vi "Relay_On_While_Running.vi"() -> ()   [LabVIEW 2022 SP3]
uses:
  <vilib>/Instr/_visa.llb/VISA Configure Serial Port (Instr).vi
panel:
  out "Controller Feedback":string
  out "Command Sent":string
  in  "VISA resource name":refnum<visa-resource-name>
  in  "Left":bool
  in  "Down":bool
  in  "Up":bool
  in  "Right":bool
  in  "Adjustor Number":dbl format="%0#3_4p"
  in  "Emergency Stop":bool
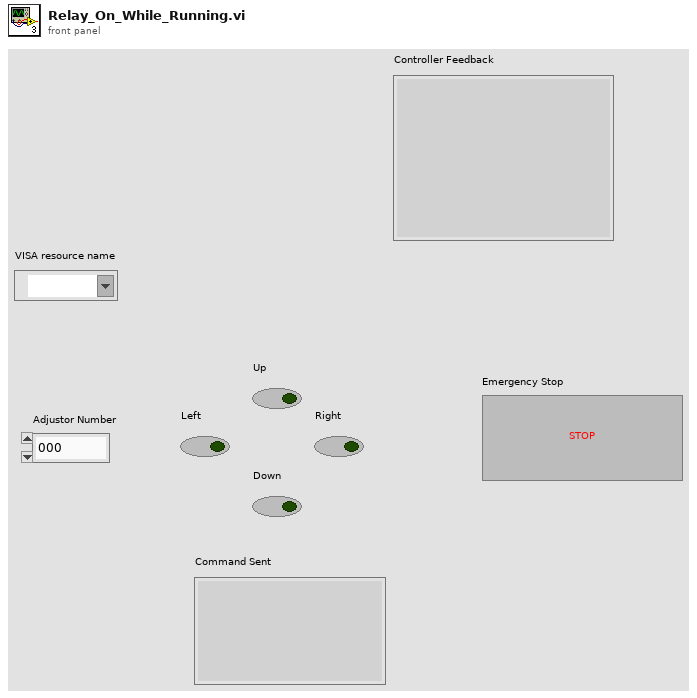
[diagram p1: front panel]
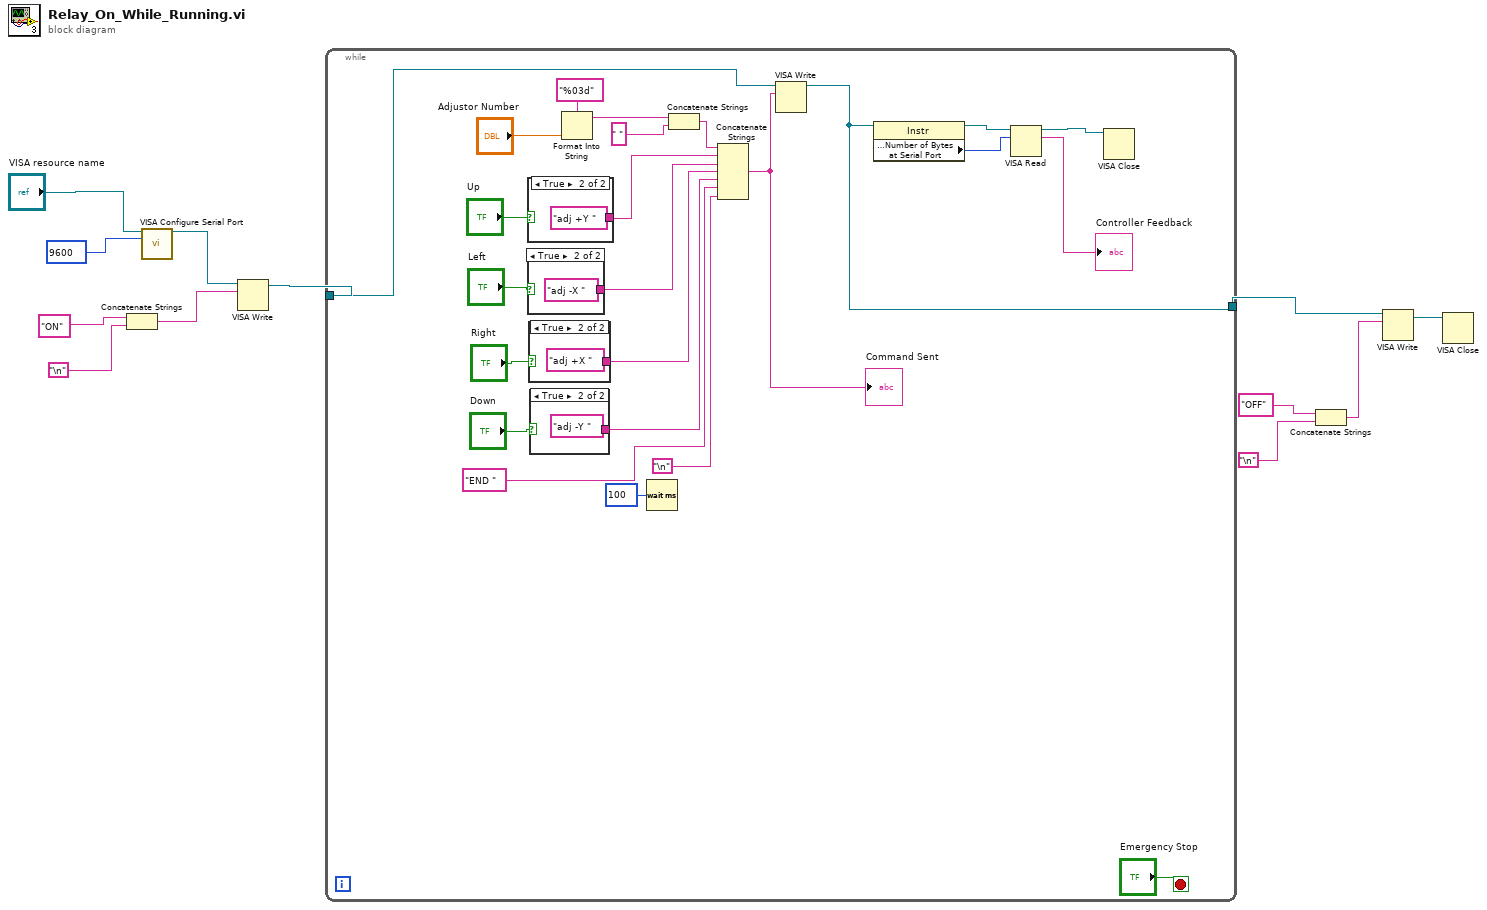
[diagram p0: block diagram]
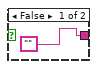
[diagram p2: hidden frame]
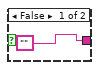
[diagram p3: hidden frame]
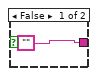
[diagram p4: hidden frame]
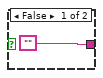
[diagram p5: hidden frame]
diagram:
  n1 = Concatenate Strings("ON", "\n") -> (w6:string)
  n2 = call-poly "VISA Configure Serial Port"("VISA resource name"="VISA resource name", "baud rate (9600)"=u32 9600) -> ("VISA resource name out"=w2:refnum<visa-resource-name>)  [unwired: 12 in, 1 out]
  n3 = VISA Write(VISA resource name=w2, write buffer=w6) -> (VISA resource name out=w1:refnum<visa-resource-name>)  [unwired: 1 in, 2 out]
  n4 = while {
    tunnel: w1 -> [w26]
    tunnel: [w16] -> w11
    stop <- "Emergency Stop" stop-if-true
    n5 = case shown="True" "Up" {
      tunnel: ["" "adj +Y "] -> w30
      frame False {
      }
      frame True {
      }
    }
    n6 = case shown="True" "Left" {
      tunnel: ["" "adj -X "] -> w29
      frame False {
      }
      frame True {
      }
    }
    n7 = case shown="True" "Right" {
      tunnel: ["" "adj +X "] -> w28
      frame False {
      }
      frame True {
      }
    }
    n8 = case shown="True" "Down" {
      tunnel: ["" "adj -Y "] -> w27
      frame False {
      }
      frame True {
      }
    }
    n9 = Format Into String(format string="%03d", "Adjustor Number") -> (resulting string=w14:string)  [unwired: 2 in, 1 out]
    n10 = Wait (ms)(milliseconds to wait=u32 100) -> ()  [unwired: 1 out]
    n11 = Concatenate Strings(w14, " ") -> (w23:string)
    n12 = Concatenate Strings(w23, w30, w29, w28, w27, "END ", "\n") -> (w25:string)
    "Command Sent" <- w25
    n13 = VISA Write(VISA resource name=w26, write buffer=w25) -> (VISA resource name out=w16:refnum<visa-resource-name>)  [unwired: 1 in, 2 out]
    n14 = property class="Instr"(reference=w16) -> (reference out=w20:refnum<visa-resource-name>, "Serial Settings:Number of Bytes at Serial Port"=w19:u32)  [unwired: 1 in, 1 out]
    n15 = VISA Read(VISA resource name=w20, byte count=w19) -> (VISA resource name out=w17:refnum<visa-resource-name>, read buffer=→"Controller Feedback":string)  [unwired: 1 in, 2 out]
    n16 = VISA Close(VISA resource name=w17) -> ()  [unwired: 1 in, 1 out]
  }
  n17 = Concatenate Strings("OFF", "\n") -> (w7:string)
  n18 = VISA Write(VISA resource name=w11, write buffer=w7) -> (VISA resource name out=w10:refnum<visa-resource-name>)  [unwired: 1 in, 2 out]
  n19 = VISA Close(VISA resource name=w10) -> ()  [unwired: 1 in, 1 out]
